vi "Cell Color Test.vi"() -> ()   [LabVIEW 2016]
uses:
  <vilib>/Utility/miscctls.llb/LVRowAndColumnTypeDef.ctl
panel:
  out "PDP Currents":string[][](table)
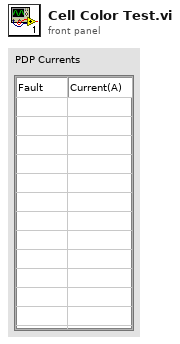
[diagram p1: front panel]
types:
  T1 = typedef "LVRowAndColumnTypeDef.ctl" = cluster{"Row":i32, "Column":i32}
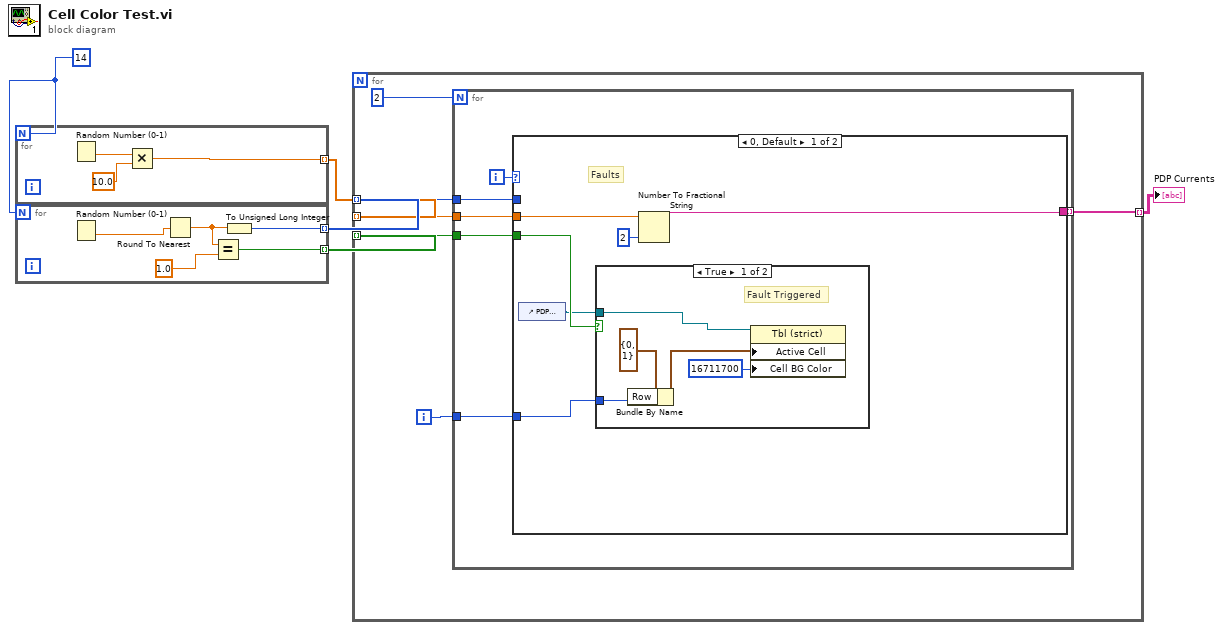
[diagram p0: block diagram]
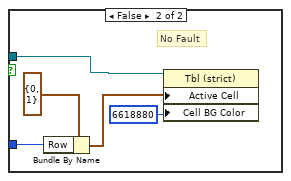
[diagram p2: hidden frame]
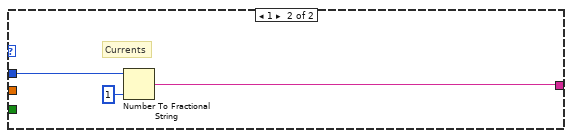
[diagram p3: hidden frame]
diagram:
  w5 = 14
  n1 = for {
    N: w5 -> [_]
    tunnel: [w6] -> w3 mode=indexing
    n2 = Random Number (0-1)() -> (number: 0 to 1=w8:dbl)
    n3 = Multiply(x=w8, y=10.0) -> (x*y=w6:dbl)
  }
  n4 = for {
    N: w5 -> [_]
    tunnel: [w12] -> w4 mode=indexing
    tunnel: [w9] -> w2 mode=indexing
    n5 = Random Number (0-1)() -> (number: 0 to 1=w13:dbl)
    n6 = Round To Nearest(number=w13) -> (nearest integer value=w10:dbl)
    n7 = Equal?(x=w10, y=1.0) -> (x = y?=w9:bool)
    n8 = To Unsigned Long Integer(number=w10) -> (unsigned 32bit integer=w12:u32)
  }
  n9 = for {
    tunnel: w4 -> [w19] mode=indexing
    tunnel: w3 -> [w17] mode=indexing
    tunnel: [w18] -> w1 mode=indexing
    tunnel: w2 -> [w15] mode=indexing
    i -> [w14]
    n10 = for {
      N: 2 -> [_]
      tunnel: [w24] -> w18 mode=indexing
      tunnel: w19 -> [w25]
      tunnel: w17 -> [w22]
      tunnel: w15 -> [w21]
      tunnel: w14 -> [w20]
      i -> [w23]
      n11 = case shown="0, Default" w23 {
        tunnel: w25 -> [_ w44]
        tunnel: [w30 w43] -> w24
        tunnel: w22 -> [w31 _]
        tunnel: w21 -> [w27 _]
        tunnel: w20 -> [w28 _]
        frame 0, Default {
          # "Faults"
          n12 = control-ref of="PDP Currents"() -> (w26:refnum<vi>)
          n13 = case shown="True" w27 {
            tunnel: w28 -> [w35 w38]
            tunnel: w26 -> [w32 w37]
            frame True {
              # "Fault Triggered"
              n14 = Bundle By Name(cluster=T1 {"Row"=0, "Column"=1} ("Active Cell:Active Cell"), "Row"=w35) -> (w33:T1)
              n15 = property class="Tbl (strict)"(reference=w32, "Active Cell"=w33, "Cell BG Color"=u32 16711700 ("Active Cell:Cell Background Color")) -> ()  [unwired: 1 in, 2 out]
            }
            frame False {
              # "No Fault"
              n16 = Bundle By Name(cluster=T1 {"Row"=0, "Column"=1} ("Active Cell:Active Cell"), "Row"=w38) -> (w39:T1)
              n17 = property class="Tbl (strict)"(reference=w37, "Active Cell"=w39, "Cell BG Color"=u32 6618880 ("Active Cell:Cell Background Color")) -> ()  [unwired: 1 in, 2 out]
            }
          }
          n18 = Number To Fractional String(number=w31, precision (6)=i16 2) -> (F-format string=w30:string)  [unwired: 2 in]
        }
        frame 1 {
          # "Currents"
          n19 = Number To Fractional String(number=w44, precision (6)=i16 1) -> (F-format string=w43:string)  [unwired: 2 in]
        }
      }
    }
  }
  "PDP Currents" <- w1
